vi "OP400ZP_prep bdd datadyn.vi"(8 "tabin":string[](array[string]), 11 "StrData":T1={"Chaîne"="20.0", "Chaîne"="22.0", "Chaîne"="3560", "Chaîne"="3561", "Chaîne"="25.0", "Chaîne"="2.0", "Chaîne"=" 1.0", "Chaîne 2"=" 1.0"}) -> (0 "tabout":string[](array[string]))   [LabVIEW 2020]
uses:
  OP400ZP_selectdata.ctl
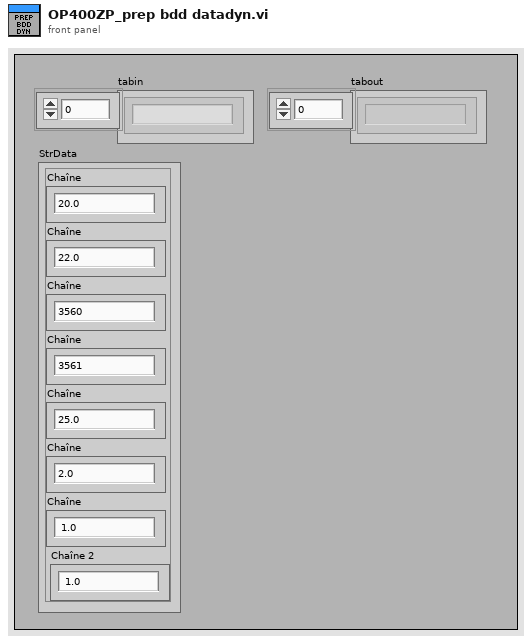
[diagram p1: front panel]
types:
  T1 = cluster{"Chaîne":string, "Chaîne":string, "Chaîne":string, "Chaîne":string, "Chaîne":string, "Chaîne":string, "Chaîne":string, "Chaîne 2":string}
  T2 = typedef "OP400ZP_selectdata.ctl" = u16
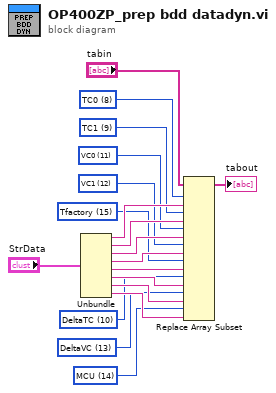
[diagram p0: block diagram]
diagram:
  w1 = T2 14 items=["IdOp400", "SN", "Type", "DateStart", "OCV", "ACIR", "InsuP", "InsuN", "TC0", "TC1", "DeltaTC", "VC0", "VC1", "DeltaVC", "MCU", "Tfactory", "RefLimite", "IniFileVers", "SoftVers", "ImageVers", "Pass", "Operateur", "TempsTest"] ("Menu déroulant")
  w2 = T2 13 items=["IdOp400", "SN", "Type", "DateStart", "OCV", "ACIR", "InsuP", "InsuN", "TC0", "TC1", "DeltaTC", "VC0", "VC1", "DeltaVC", "MCU", "Tfactory", "RefLimite", "IniFileVers", "SoftVers", "ImageVers", "Pass", "Operateur", "TempsTest"] ("Menu déroulant")
  w3 = T2 10 items=["IdOp400", "SN", "Type", "DateStart", "OCV", "ACIR", "InsuP", "InsuN", "TC0", "TC1", "DeltaTC", "VC0", "VC1", "DeltaVC", "MCU", "Tfactory", "RefLimite", "IniFileVers", "SoftVers", "ImageVers", "Pass", "Operateur", "TempsTest"] ("Menu déroulant")
  w4 = T2 15 items=["IdOp400", "SN", "Type", "DateStart", "OCV", "ACIR", "InsuP", "InsuN", "TC0", "TC1", "DeltaTC", "VC0", "VC1", "DeltaVC", "MCU", "Tfactory", "RefLimite", "IniFileVers", "SoftVers", "ImageVers", "Pass", "Operateur", "TempsTest"] ("Menu déroulant")
  w5 = T2 12 items=["IdOp400", "SN", "Type", "DateStart", "OCV", "ACIR", "InsuP", "InsuN", "TC0", "TC1", "DeltaTC", "VC0", "VC1", "DeltaVC", "MCU", "Tfactory", "RefLimite", "IniFileVers", "SoftVers", "ImageVers", "Pass", "Operateur", "TempsTest"] ("Menu déroulant")
  w6 = T2 11 items=["IdOp400", "SN", "Type", "DateStart", "OCV", "ACIR", "InsuP", "InsuN", "TC0", "TC1", "DeltaTC", "VC0", "VC1", "DeltaVC", "MCU", "Tfactory", "RefLimite", "IniFileVers", "SoftVers", "ImageVers", "Pass", "Operateur", "TempsTest"] ("Menu déroulant")
  w7 = T2 9 items=["IdOp400", "SN", "Type", "DateStart", "OCV", "ACIR", "InsuP", "InsuN", "TC0", "TC1", "DeltaTC", "VC0", "VC1", "DeltaVC", "MCU", "Tfactory", "RefLimite", "IniFileVers", "SoftVers", "ImageVers", "Pass", "Operateur", "TempsTest"] ("Menu déroulant")
  w8 = T2 8 items=["IdOp400", "SN", "Type", "DateStart", "OCV", "ACIR", "InsuP", "InsuN", "TC0", "TC1", "DeltaTC", "VC0", "VC1", "DeltaVC", "MCU", "Tfactory", "RefLimite", "IniFileVers", "SoftVers", "ImageVers", "Pass", "Operateur", "TempsTest"] ("Menu déroulant")
  n1 = Unbundle("StrData") -> ("Chaîne"=w17:string, "Chaîne"=w15:string, "Chaîne"=w14:string, "Chaîne"=w13:string, "Chaîne"=w12:string, "Chaîne"=w11:string, "Chaîne"=w10:string, "Chaîne 2"=w9:string)
  n2 = Replace Array Subset(array="tabin", new element #1=w17, index #1=w8, new element #2=w15, index #2=w7, new element #3=w14, index #3=w6, new element #4=w13, index #4=w5, new element #5=w12, index #5=w4, new element #6=w11, index #6=w3, new element #7=w10, index #7=w2, new element #8=w9, index #8=w1) -> (→"tabout":string[])
